vi "VIRef_Find Largest Decoration.vi"(8 "Error":errorcluster, 9 "Decoration index":i32, 11 "VI's Ref":refnum<vi>) -> (0 "Error Out":errorcluster, 1 "Found":bool, 2 "Decor Refnum Out":refnum<vi>, 3 "Calling VI's Ref Out":refnum<vi>)   [LabVIEW 2020]
doc: "Finds the largest decoration in a vis Front panel"
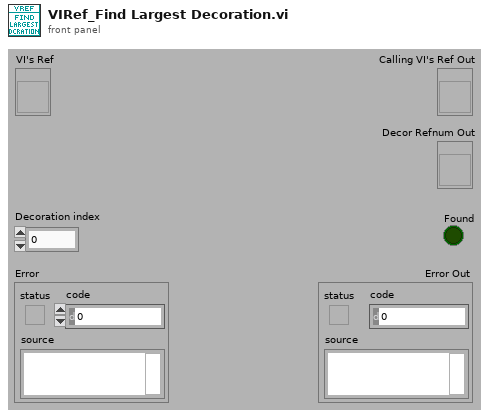
[diagram p1: front panel]
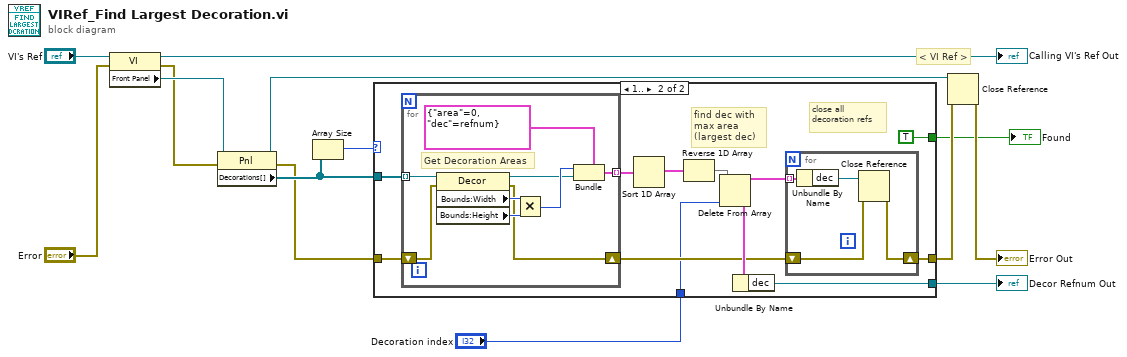
[diagram p0: block diagram]
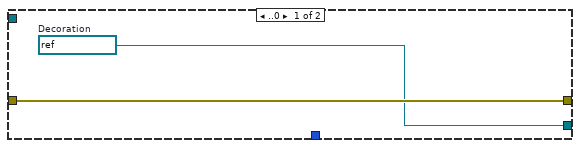
[diagram p2: hidden frame]
diagram:
  # "< VI Ref >"
  n1 = property on="Property Node" class="VI"(reference="VI's Ref", error in="Error") -> (reference out=→"Calling VI's Ref Out":refnum<vi>, error out=w4:errorcluster, "Front Panel"=w8:refnum<vi>)
  n2 = property on="Property Node" class="Pnl"(reference=w8, error in=w4) -> (reference out=w6:refnum<vi>, error out=w3:errorcluster, "Decorations[]"=w9:refnum<vi>[])
  n3 = Array Size(array=w9) -> (size(s)=w10:i32)
  n4 = case shown="1.." w10 {
    tunnel: w3 -> [w16 w28]
    tunnel: [w15 w18] -> w12
    tunnel: w9 -> [_ w26]
    tunnel: [w16 w23] -> w14
    tunnel: "Decoration index" -> [_ w19]
    tunnel: [_ TRUE] -> w1
    frame ..0 {
      w15 = refnum<vi> refnum  # Decoration
    }
    frame 1.. {
      # "close all  decoration refs"
      # "find dec with max area (largest dec)"
      n5 = for {
        tunnel: w26 -> [w37] mode=indexing
        shift-right: [w33] -> w24
        shift-left: w28 -> [w34]
        tunnel: [w30] -> w22 mode=indexing
        # "Get Decoration Areas"
        n6 = property class="Decor"(reference=w37, error in=w34) -> (reference out=w31:refnum<vi>, error out=w33:errorcluster, "Bounds:Width"=w36:u32, "Bounds:Height"=w35:u32)
        n7 = Multiply(x=w36, y=w35) -> (x*y=w32:u32)
        n8 = Bundle(cluster=cluster{"area":u32, "dec":refnum<vi>} {"area"=0, "dec"=refnum}, "area"=w32, "dec"=w31) -> (w30:cluster{"area":u32, "dec":refnum<vi>})
      }
      n9 = Sort 1D Array(array=w22) -> (sorted array=w21:cluster{"area":u32, "dec":refnum<vi>}[])
      n10 = Reverse 1D Array(array=w21) -> (reversed array=w20:cluster{"area":u32, "dec":refnum<vi>}[])
      n11 = Delete From Array(array=w20, index=w19) -> (deleted portion=w27:cluster{"area":u32, "dec":refnum<vi>}, array with subset deleted=w25:cluster{"area":u32, "dec":refnum<vi>}[])  [unwired: 1 in]
      n12 = Unbundle By Name(w27) -> ("dec"=w18:refnum<vi>)
      n13 = for {
        tunnel: w25 -> [w41] mode=indexing
        shift-right: [w39] -> w23
        shift-left: w24 -> [w40]
        n14 = Unbundle By Name(w41) -> ("dec"=w38:refnum<vi>)
        n15 = Close Reference(reference=w38, error in (no error)=w40) -> (error out=w39:errorcluster)
      }
    }
  }
  "Decor Refnum Out" <- w12
  "Found" <- w1
  n16 = Close Reference(reference=w6, error in (no error)=w14) -> (error out=→"Error Out":errorcluster)
